vi "Event Generate.vi"(7 "Priority Message":bool, 8 "error in":errorcluster, 11 "Event Type":T1) -> (0 "error out":errorcluster)   [LabVIEW 2020, in "GUI.lvlib"]
doc: "ENqueue a message for this component."
uses:
  GUI.lvlib
  Event Type.ctl
  Event FGV Actions.ctl
  <vilib>/event_ctls.llb/usereventprio.ctl
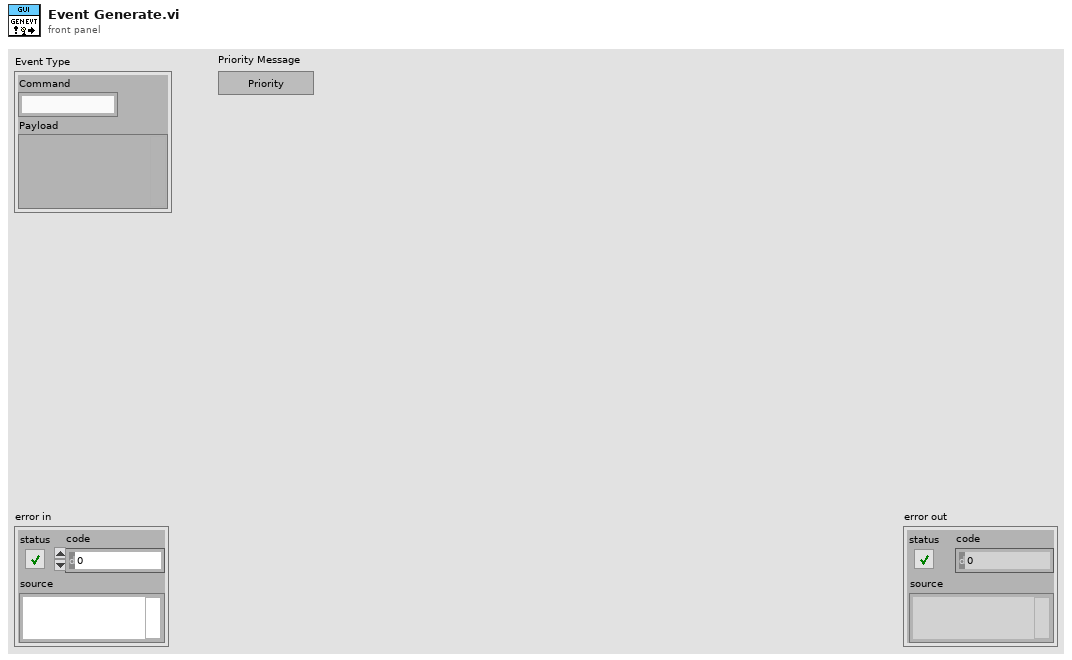
[diagram p1: front panel]
types:
  T1 = typedef "GUI.lvlib/Event Type.ctl" = cluster{"Command":string, "Payload":variant}
  T2 = typedef "GUI.lvlib/Event FGV Actions.ctl" = enum16{"Get", "Create", "Destroy"}
  T3 = typedef "usereventprio.ctl" = enum32{"high priority", "normal priority"}
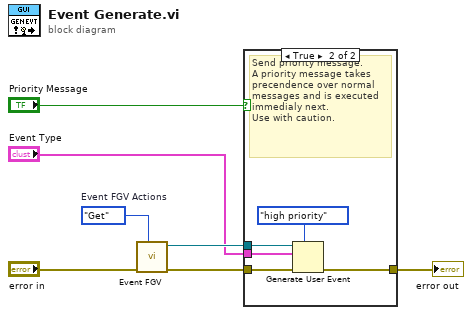
[diagram p0: block diagram]
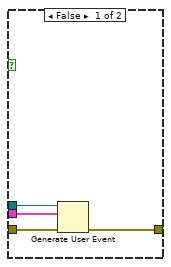
[diagram p2: hidden frame]
diagram:
  w5 = Event_FGV_Actions."Get"  # Event FGV Actions
  n1 = call "Event FGV.vi"("Event FGV Actions"=w5, "error in"="error in") -> ("error out"=w6:errorcluster, "API Event Message"=w3:refnum<user-event>)  [unwired: 7 in, 1 out]
  n2 = case shown="True" "Priority Message" {
    tunnel: w6 -> [w11 w16]
    tunnel: [w10 w15] -> w4
    tunnel: w3 -> [w9 w14]
    tunnel: "Event Type" -> [w8 w13]
    frame False {
      n3 = Generate User Event(user event=w9, event data cluster=w8, error in=w11) -> (error out=w10:errorcluster)  [unwired: 1 in, 1 out]
    }
    frame True {
      # "Send priority message.\nA priority message takes precendence over normal messages and is executed immedialy next.\nUse with caution."
      n4 = Generate User Event(priority (normal)=usereventprio."high priority", user event=w14, event data cluster=w13, error in=w16) -> (error out=w15:errorcluster)  [unwired: 1 out]
    }
  }
  "error out" <- w4
